vi "Flush Analog Acquisition FIFO.vi"(8 "error in":errorcluster, 11 "FPGA VI Reference":refnum<k20>) -> (0 "error out":errorcluster, 2 "Analog Data":sgl[][](array[numeric]), 3 "FPGA VI Reference":refnum<k20>)   [LabVIEW 2020]
uses:
  <vilib>/Utility/error.llb/Error Cluster From Error Code.vi
  <vilib>/rvi/errors/niLvFpgaAdjustHostInterfaceError.vi
  <vilib>/rvi/interface/nirviReadWriteControl/nirviReadWriteControl.xnode
  <vilib>/rvi/interface/nirviMethod/nirviMethod.xnode
  <vilib>/FPGAPlugInAG/Dynamic/niLvFpga_ReadFifo_Dynamic.vi
  <vilib>/rvi/errors/niLvFpgaMergeErrorWithErrorCode.vi
  NiFpgaLv.dll
  <vilib>/rvi/interface/Simulation/niFpgaSimulationCallBeginRW.vi
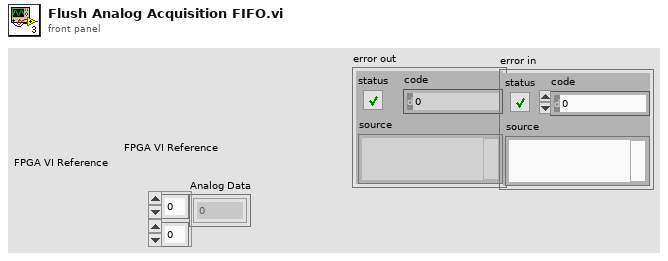
[diagram p1: front panel]
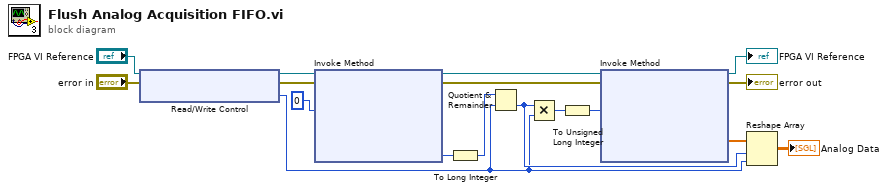
[diagram p0: block diagram]
diagram:
  n1 = xnode "Read/Write Control"("FPGA VI Reference In"="FPGA VI Reference", "error in"="error in") -> ("FPGA VI Reference Out"=w13:refnum<k20>, "error out"=w7:errorcluster, "Analog Channel Count"=w1:i32)
  n2 = xnode "Invoke Method"("FPGA VI Reference In"=w13, "error in"=w7, "Number of Elements"=u32 0) -> ("FPGA VI Reference Out"=w11:refnum<k20>, "error out"=w6:errorcluster, "Elements Remaining"=w9:u32)  [unwired: 1 in, 1 out]
  n3 = To Long Integer(number=w9) -> (32bit integer=w10:i32)
  n4 = Quotient & Remainder(x=w10, y=w1) -> (floor(x/y)=w14:i32)  [unwired: 1 out]
  n5 = Multiply(x=w14, y=w1) -> (x*y=w15:i32)
  n6 = To Unsigned Long Integer(number=w15) -> (unsigned 32bit integer=w16:u32)
  n7 = xnode "Invoke Method"("FPGA VI Reference In"=w11, "error in"=w6, "Number of Elements"=w16) -> ("FPGA VI Reference Out"=→"FPGA VI Reference":refnum<k20>, "error out"=→"error out":errorcluster, "Data"=w12:sgl[])  [unwired: 1 in, 1 out]
  n8 = Reshape Array(w12, w14, w1) -> (→"Analog Data":sgl[][])
